vi "_Add Row.vi"(8 "error in":errorcluster, 10 "RowIndex":i32, 11 "Worksheet in":refnum<k24>) -> (0 "error out":errorcluster, 2 "Row":refnum<k24>, 3 "Worksheet out":refnum<k24>)   [LabVIEW 2021, in "Open Xml.lvlib"]
uses:
  Open Xml.lvlib
  D:/git/Open-Xml-LabVIEW/dll/DocumentFormat.OpenXml.dll
  dll/DocumentFormat.OpenXml.dll
  D:/git/Open-Xml-LabVIEW/dll/DocumentFormat.OpenXml.Framework.dll
  dll/DocumentFormat.OpenXml.Framework.dll
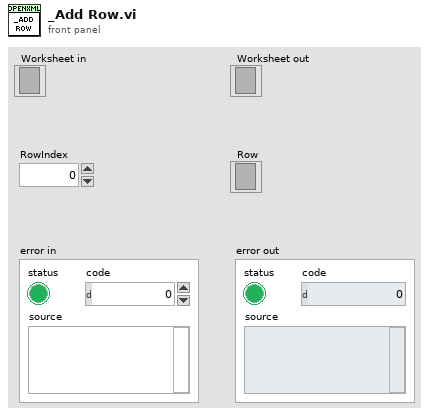
[diagram p1: front panel]
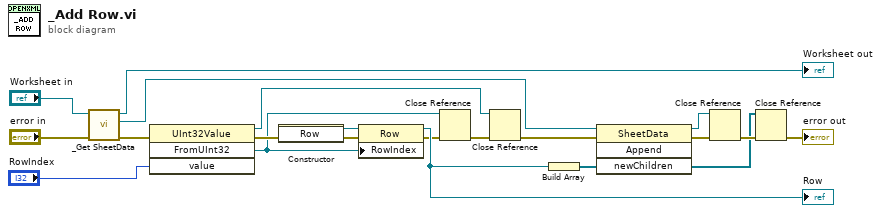
[diagram p0: block diagram]
diagram:
  n1 = call "_Get SheetData.vi"("error in"="error in", "Worksheet in"="Worksheet in") -> ("error out"=w7:errorcluster, "SheetData"=w15:refnum<k24>, "Worksheet out"=→"Worksheet out":refnum<k24>)  [unwired: 7 in]
  n2 = invoke class="UInt32Value" method="FromUInt32"(error in=w7, "value"="RowIndex") -> (reference out=w8:refnum<k24>, error out=w6:errorcluster, "FromUInt32"=w1:refnum<k24>)  [unwired: 2 in, 1 out]
  n3 = constructor class="Row"(error in=w6) -> (reference out=w12:refnum<k24>, error out=w5:errorcluster)  [unwired: 2 in, 1 out]
  n4 = property class="Row"(reference=w12, error in=w5, "RowIndex"=w1) -> (reference out=w20:refnum<k24>, error out=w10:errorcluster)
  "Row" <- w20
  n5 = Close Reference(reference=w1, error in (no error)=w10) -> (error out=w2:errorcluster)
  n6 = Close Reference(reference=w8, error in (no error)=w2) -> (error out=w9:errorcluster)
  n7 = Build Array(w20) -> (w18:refnum<k24>[])
  n8 = invoke class="SheetData" method="Append"(reference=w15, error in=w9, "newChildren"=w18) -> (reference out=w17:refnum<k24>, error out=w16:errorcluster, "newChildren"=w3:refnum<k24>[])  [unwired: 1 in, 1 out]
  n9 = Close Reference(reference=w17, error in (no error)=w16) -> (error out=w19:errorcluster)
  n10 = Close Reference(reference=w3, error in (no error)=w19) -> (error out=→"error out":errorcluster)
